vi "产品删除.vi"(8 "error in (no error)":errorcluster caption="错误输入（无错误）") -> (0 "error in (no error) 2":errorcluster caption="错误输入（无错误）")   [LabVIEW 2017]
uses:
  Picture/SaveButtom.ctl
  Global System.vi
panel:
  out "路径输出":path
  out "添加的路径":path
  in  "Vision Paramter Save Buttom":T1
  out "system time":string
  in  "取消按钮":bool
  in  "执行按钮":bool
  in  "原有产品型号":string(combo)
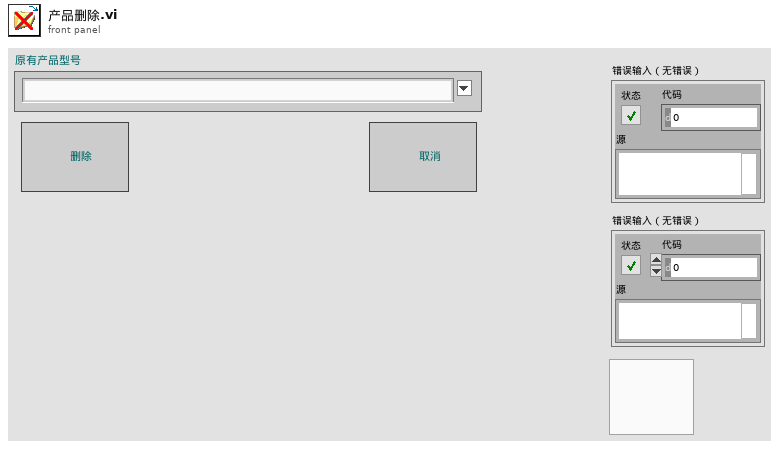
[diagram p1: front panel]
types:
  T1 = typedef "SaveButtom.ctl" = bool
  T2 = cluster{"index":i32, "this vi":refnum<vi>, "error out":errorcluster}
  T3 = cluster{"master data":string, "priority":u16, "secondary data":string[]}
  T4 = cluster{"case name":string[], "queue array":refnum<queue>[]}
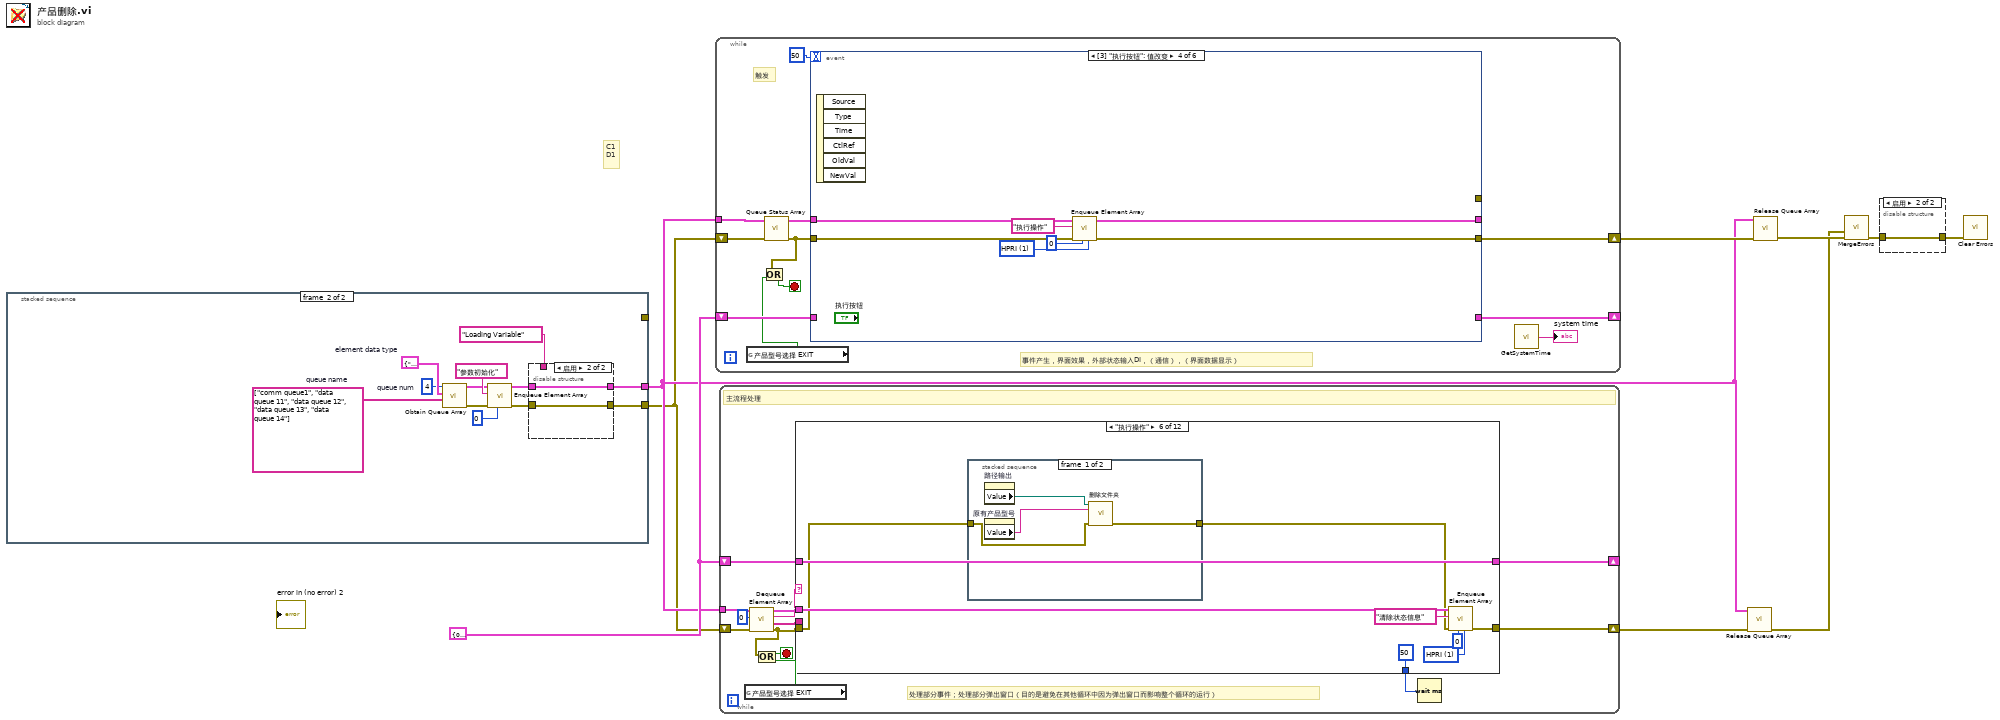
[diagram p0: block diagram]
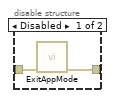
[diagram p2: hidden frame]
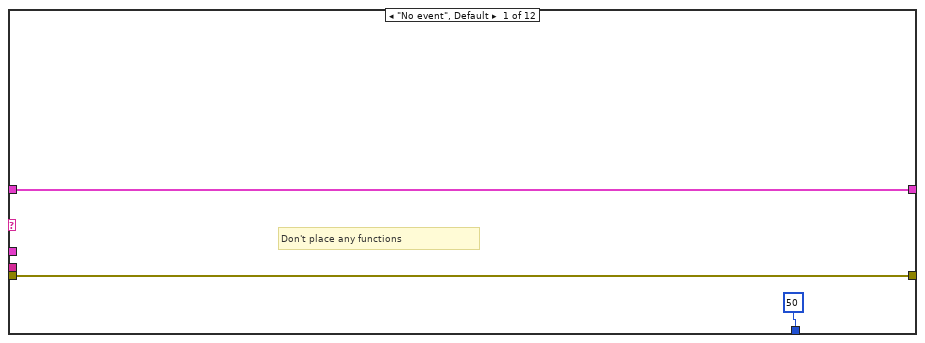
[diagram p3: hidden frame]
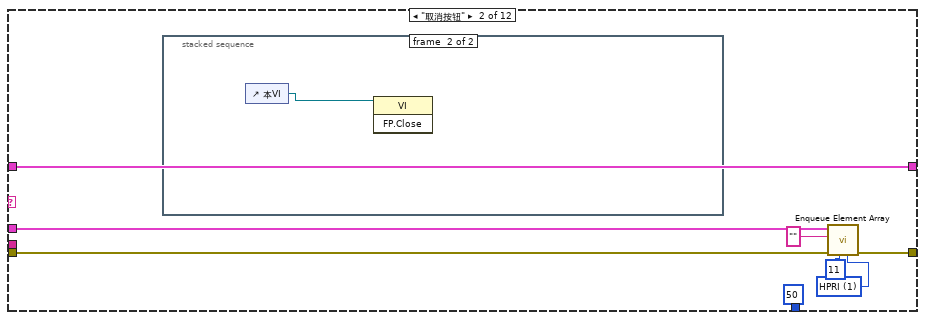
[diagram p4: hidden frame]
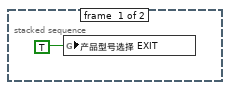
[diagram p5: hidden frame]
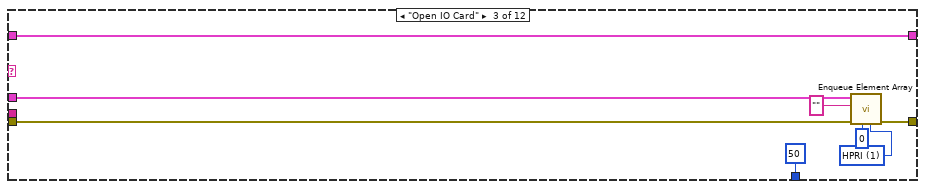
[diagram p6: hidden frame]
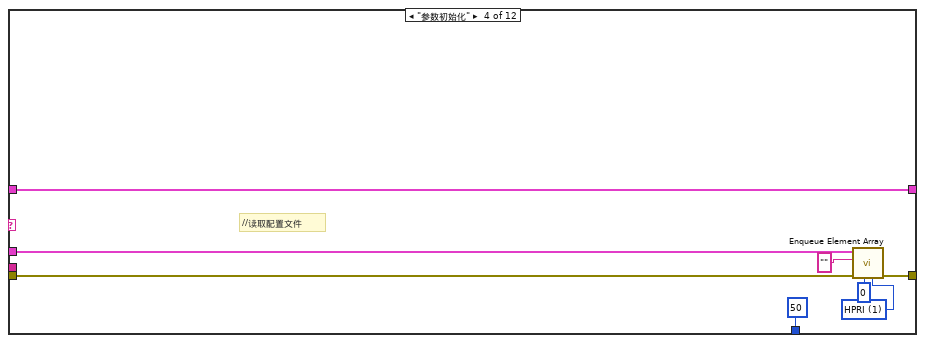
[diagram p7: hidden frame]
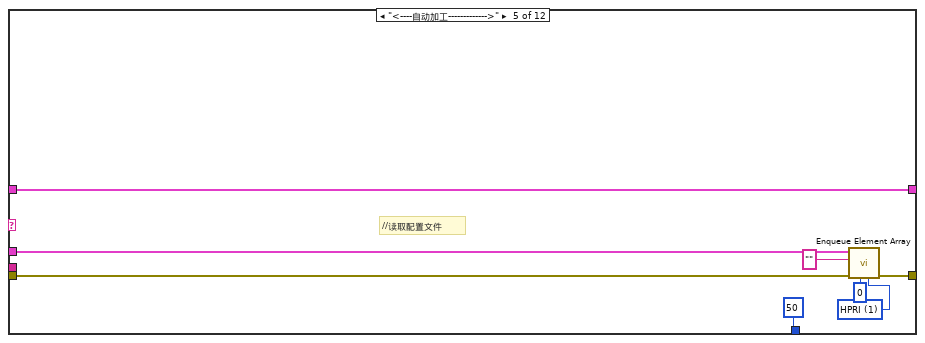
[diagram p8: hidden frame]
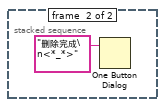
[diagram p9: hidden frame]
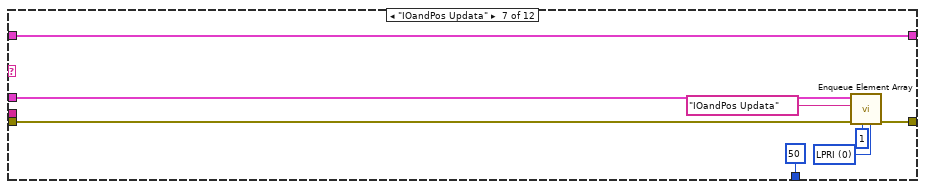
[diagram p10: hidden frame]
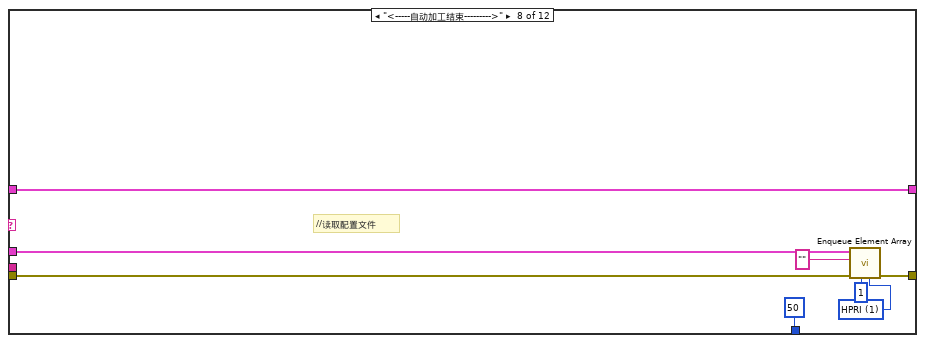
[diagram p11: hidden frame]
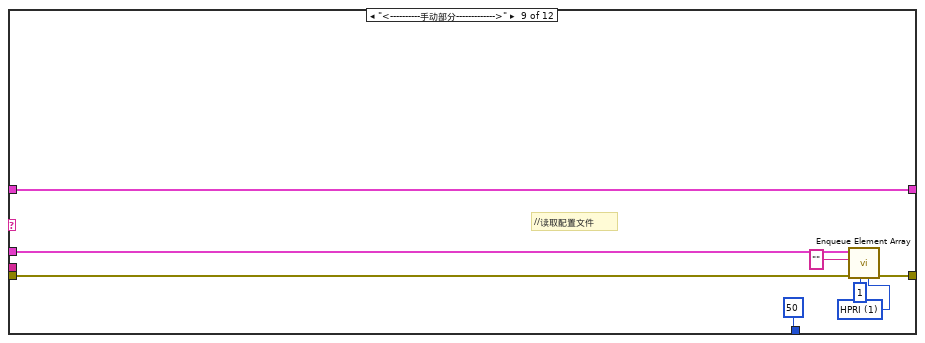
[diagram p12: hidden frame]
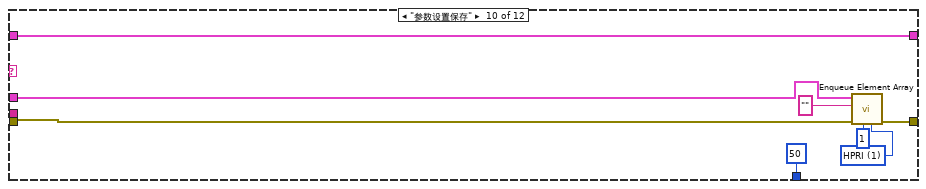
[diagram p13: hidden frame]
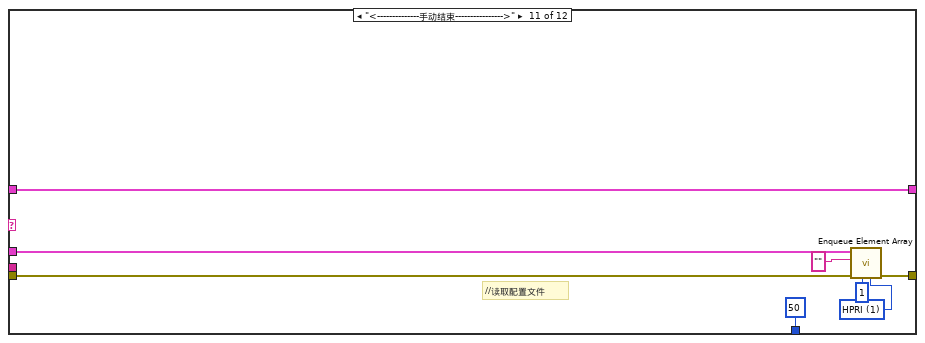
[diagram p14: hidden frame]
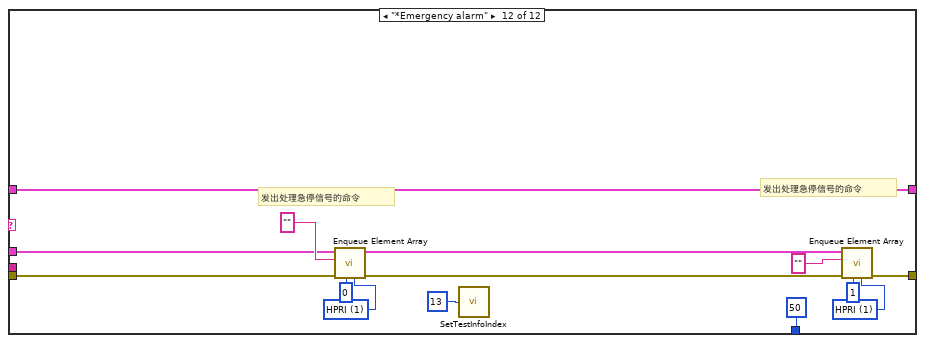
[diagram p15: hidden frame]
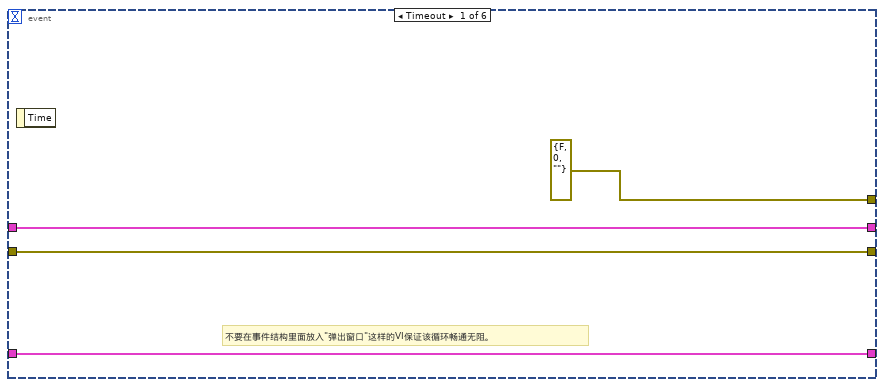
[diagram p16: hidden frame]
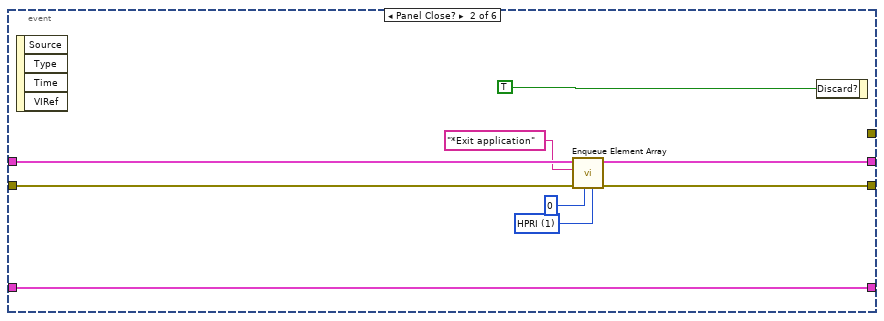
[diagram p17: hidden frame]
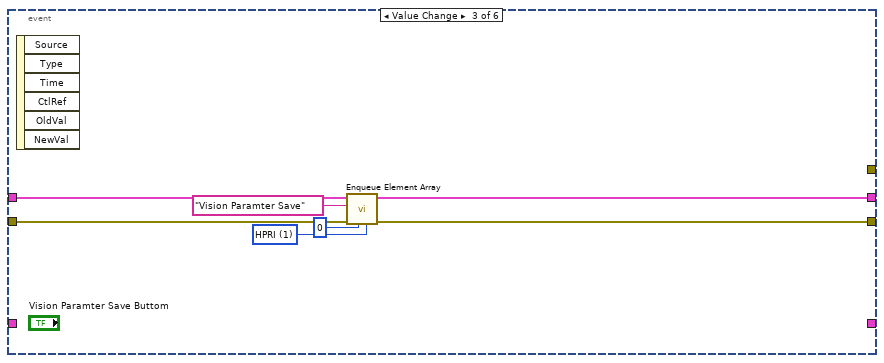
[diagram p18: hidden frame]
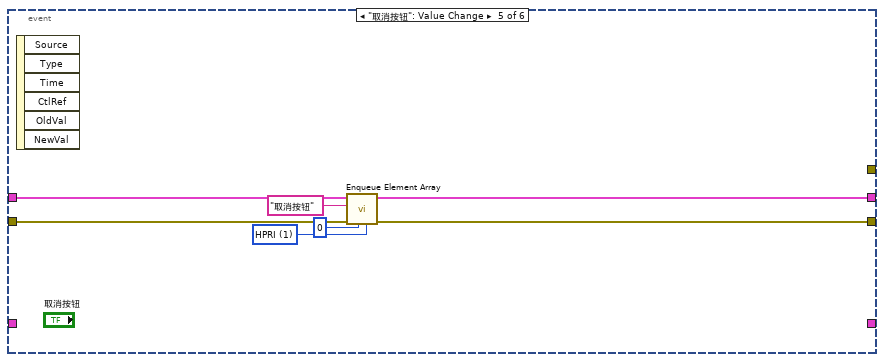
[diagram p19: hidden frame]
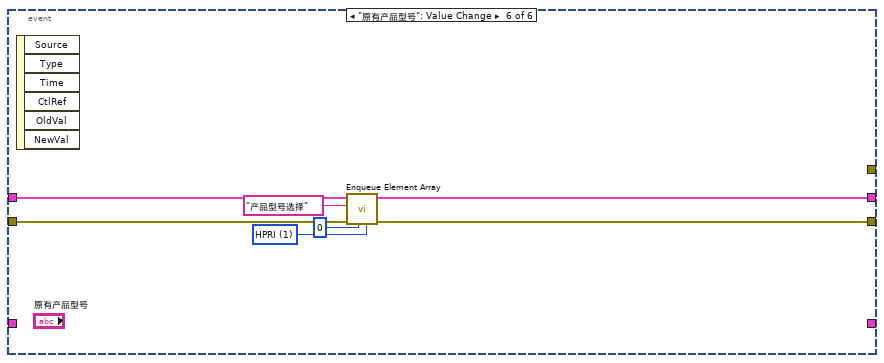
[diagram p20: hidden frame]
diagram:
  w5 = T2 {"index"=0, "this vi"=refnum, "error out"={"status"=FALSE, "code"=0, "source"=""}} ("parameter buffer")
  # "C1\nD1"
  n1 = stacked-sequence {
    tunnel: [w12 _] -> _
    tunnel: [_ w18] -> w1
    tunnel: [_ w17] -> w2
    frame #0 {
      n2 = global write "Global System.vi" "A1 EXIT"(FALSE ("A1 EXIT")) -> ()
      n3 = global read "Global System.vi" "ref path"() -> (w13:path)
      n4 = Build Path(base path=w13, name or relative path="Template Program" ("名称或相对路径")) -> (appended path=w15:path)
      "添加的路径" <- w15
      n5 = List Folder(path=w15) -> (path out=→"路径输出":path, folder names=w16:string[], error out=w12:errorcluster)  [unwired: 3 in, 1 out]
      n6 = property on="原有产品型号" class="CmbBox"("Strings[]"=w16) -> ()  [unwired: 2 in, 2 out]
    }
    frame #1 {
      w26 = string[] ["comm queue1", "data queue 11", "data queue 12", "data queue 13", "data queue 14"]  # queue name
      w27 = 4  # queue num
      w28 = T3 {"master data"="", "priority"=0, "secondary data"=[]}  # element data type
      n7 = call "Obtain Queue Array.vi"("queue name"=w26, "element data type"=w28, "queue num"=w27) -> ("error out"=w22:errorcluster, "queue out"=w23:T4)  [unwired: 2 in, 1 out]
      n8 = call "Enqueue Element Array.vi"("queue index"=0, "error in"=w22, "master data"="参数初始化", "queue in"=w23) -> ("error out"=w21:errorcluster, "queue out"=w20:T4)  [unwired: 6 in]
      n9 = disable-structure shown="启用" {
        disable-tunnel: w21 -> [w34 w35]
        disable-tunnel: w20 -> [w33 w36]
        disable-tunnel: "Loading Variable" ("master data") -> [w32 _]
        disable-tunnel: [w30 w35] -> w18
        disable-tunnel: [w29 w36] -> w17
        frame Disabled {
          n10 = call "Enqueue Element Array.vi"("queue index"=12, "error in"=w34, "master data"=w32, "queue in"=w33) -> ("error out"=w30:errorcluster, "queue out"=w29:T4)  [unwired: 6 in]
        }
        frame Enabled {
        }
      }
    }
  }
  n11 = while {
    shift-right: [w40] -> w6
    shift-left: w1 -> [w44]
    shift-right: [w42] -> _
    shift-left: w5 -> [w43]
    tunnel: w2 -> [w46]
    stop <- w37 stop-if-true
    # "触发"
    # "事件产生，界面效果，外部状态输入DI，（通信），（界面数据显示）"
    n12 = global read "Global System.vi" "产品型号选择 EXIT"() -> (w38:bool)
    n13 = call "Queue Status Array.vi"("error in (no error)"=w44, "queue in"=w46) -> ("error out"=w39:errorcluster, "queue out"=w41:T4)  [unwired: 4 in]
    n14 = Or(x=w39, y=w38) -> (x .or. y?=w37:bool)
    n15 = event shown="[3] \"执行按钮\": 值改变" {
      selector: _ -> [_ _ _ _ _ _]
      dyn-events: _ -> [_ _ _ _ _ _]
      timeout: 50 -> [_ _ _ _ _ _]
      tunnel: w43 -> [w51 w59 _ _ _ _]
      tunnel: [w51 w59 _ _ _ _] -> w42
      tunnel: [errorcluster {"status"=FALSE, "code"=0, "source"=""} ("error out") _ _ _ _ _] -> _
      tunnel: w41 -> [w49 w58 w64 w71 w78 w85]
      tunnel: w39 -> [w48 w57 w63 w70 w77 w84]
      tunnel: [w48 w56 w61 w68 w75 w82] -> w40
      tunnel: [w49 w55 w62 w69 w76 w83] -> _
      event Timeout {
        # "不要在事件结构里面放入\"弹出窗口\"这样的VI保证该循环畅通无阻。"
        n16 = event-data() -> ()  [unwired: 1 in, 1 out]
      }
      event Panel Close? {
        w53 = u16 1 items=["HPRI"=1, "LPRI"=0] ("priority")
        n17 = event-data() -> ()  [unwired: 1 in, 4 out]
        n18 = call "Enqueue Element Array.vi"("priority"=w53, "queue index"=0, "error in"=w57, "master data"="*Exit application", "queue in"=w58) -> ("error out"=w56:errorcluster, "queue out"=w55:T4)  [unwired: 5 in]
        n19 = event-data("Discard?"=TRUE) -> ()  [unwired: 1 in, 1 out]
      }
      event Value Change {
        w66 = u16 1 items=["HPRI"=1, "LPRI"=0] ("priority")
        n20 = event-data() -> ()  [unwired: 1 in, 6 out]
        n21 = call "Enqueue Element Array.vi"("priority"=w66, "queue index"=0, "error in"=w63, "master data"="Vision Paramter Save", "queue in"=w64) -> ("error out"=w61:errorcluster, "queue out"=w62:T4)  [unwired: 5 in]
      }
      event "执行按钮": Value Change {
        w73 = u16 1 items=["HPRI"=1, "LPRI"=0] ("priority")
        n22 = event-data() -> ()  [unwired: 1 in, 6 out]
        n23 = call "Enqueue Element Array.vi"("priority"=w73, "queue index"=0, "error in"=w70, "master data"="执行操作", "queue in"=w71) -> ("error out"=w68:errorcluster, "queue out"=w69:T4)  [unwired: 5 in]
      }
      event "取消按钮": Value Change {
        w80 = u16 1 items=["HPRI"=1, "LPRI"=0] ("priority")
        n24 = event-data() -> ()  [unwired: 1 in, 6 out]
        n25 = call "Enqueue Element Array.vi"("priority"=w80, "queue index"=0, "error in"=w77, "master data"="取消按钮", "queue in"=w78) -> ("error out"=w75:errorcluster, "queue out"=w76:T4)  [unwired: 5 in]
      }
      event "原有产品型号": Value Change {
        w87 = u16 1 items=["HPRI"=1, "LPRI"=0] ("priority")
        n26 = event-data() -> ()  [unwired: 1 in, 6 out]
        n27 = call "Enqueue Element Array.vi"("priority"=w87, "queue index"=0, "error in"=w84, "master data"="产品型号选择", "queue in"=w85) -> ("error out"=w82:errorcluster, "queue out"=w83:T4)  [unwired: 5 in]
      }
    }
    n28 = call "GetSystemTime.vi"() -> ("date/time string"=→"system time":string)  [unwired: 7 in]
  }
  n29 = while {
    shift-right: [w101] -> w4
    shift-left: w1 -> [w92]
    shift-right: [w98] -> _
    shift-left: w5 -> [w99]
    tunnel: w2 -> [w94]
    stop <- w89 stop-if-true
    # "处理部分事件；处理部分弹出窗口（目的是避免在其他循环中因为弹出窗口而影响整个循环的运行）"
    # "主流程处理"
    n30 = global read "Global System.vi" "产品型号选择 EXIT"() -> (w90:bool)
    n31 = call "Dequeue Element Array.vi"("queue in"=w94, "queue index"=0, "error in"=w92) -> ("queue out"=w97:T4, "master data"=w96:string, "secondary data"=w95:string[], "error out"=w91:errorcluster)  [unwired: 2 in, 1 out]
    n32 = Or(x=w91, y=w90) -> (x .or. y?=w89:bool)
    n33 = case shown="\"执行操作\"" w96 {
      tunnel: w97 -> [_ w111 w121 w129 w137 w141 w159 w167 w175 w183 w191 w197]
      tunnel: w91 -> [w103 w107 w117 w126 w133 w140 w154 w163 w171 w179 w187 w194]
      tunnel: [w103 w110 w120 w128 w136 w146 w158 w166 w174 w182 w190 w205] -> w101
      tunnel: [50 50 50 50 50 50 50 50 50 50 50 50] -> w100
      tunnel: w99 -> [w104 w108 w118 w123 w134 w142 w153 w164 w172 w180 w188 w203]
      tunnel: [w104 w108 w118 w123 w134 w142 w153 w164 w172 w180 w188 w203] -> w98
      tunnel: w95 -> [_ _ _ _ _ _ _ _ _ _ _ _]
      frame "No event", Default {
        # "Don't place any functions"
      }
      frame "取消按钮" {
        w105 = u16 1 items=["HPRI"=1, "LPRI"=0] ("priority")
        n34 = stacked-sequence {
          frame #0 {
            n35 = global write "Global System.vi" "产品型号选择 EXIT"(TRUE ("EXIT")) -> ()
          }
          frame #1 {
            n36 = control-ref of="本VI"() -> (w114:refnum<vi>)
            n37 = invoke class="VI" method="FP.Close"(reference=w114) -> ()  [unwired: 2 in, 3 out]
          }
        }
        n38 = call "Enqueue Element Array.vi"("priority"=w105, "queue index"=11, "error in"=w107, "master data"="" ("Element 1"), "queue in"=w111) -> ("error out"=w110:errorcluster)  [unwired: 5 in, 1 out]
      }
      frame "Open IO Card" {
        w115 = u16 1 items=["HPRI"=1, "LPRI"=0] ("priority")
        n39 = call "Enqueue Element Array.vi"("priority"=w115, "queue index"=0, "error in"=w117, "master data"="" ("Element 1"), "queue in"=w121) -> ("error out"=w120:errorcluster)  [unwired: 5 in, 1 out]
      }
      frame "参数初始化" {
        w124 = u16 1 items=["HPRI"=1, "LPRI"=0] ("priority")
        # "//读取配置文件"
        n40 = call "Enqueue Element Array.vi"("priority"=w124, "queue index"=0, "error in"=w126, "master data"="" ("Element 1"), "queue in"=w129) -> ("error out"=w128:errorcluster)  [unwired: 5 in, 1 out]
      }
      frame "<----自动加工------------->" {
        w131 = u16 1 items=["HPRI"=1, "LPRI"=0] ("priority")
        # "//读取配置文件"
        n41 = call "Enqueue Element Array.vi"("priority"=w131, "queue index"=0, "error in"=w133, "master data"="" ("Element 1"), "queue in"=w137) -> ("error out"=w136:errorcluster)  [unwired: 5 in, 1 out]
      }
      frame "执行操作" {
        w143 = u16 1 items=["HPRI"=1, "LPRI"=0] ("priority")
        n42 = stacked-sequence {
          tunnel: w140 -> [w149 _]
          tunnel: [w148 _] -> w139
          frame #0 {
            n43 = property on="路径输出" class="Path"() -> ("Value"=w151:path)  [unwired: 2 in, 2 out]
            n44 = property on="原有产品型号" class="CmbBox"() -> ("Value"=w150:string)  [unwired: 2 in, 2 out]
            n45 = call "删除文件夹.vi"("产品型号路径"=w151, "产品型号"=w150, "error in (no error)"=w149) -> ("error out"=w148:errorcluster)  [unwired: 12 in]
          }
          frame #1 {
            n46 = One Button Dialog(message="删除完成\n<*_*>" ("消息")) -> ()  [unwired: 1 in, 1 out]
          }
        }
        n47 = call "Enqueue Element Array.vi"("priority"=w143, "queue index"=0, "error in"=w139, "master data"="清除状态信息" ("Element 1"), "queue in"=w141) -> ("error out"=w146:errorcluster)  [unwired: 5 in, 1 out]
      }
      frame "IOandPos Updata" {
        w156 = u16 0 items=["HPRI"=1, "LPRI"=0] ("priority")
        n48 = call "Enqueue Element Array.vi"("priority"=w156, "queue index"=1, "error in"=w154, "master data"="IOandPos Updata", "queue in"=w159) -> ("error out"=w158:errorcluster)  [unwired: 5 in, 1 out]
      }
      frame "<-----自动加工结束--------->" {
        w161 = u16 1 items=["HPRI"=1, "LPRI"=0] ("priority")
        # "//读取配置文件"
        n49 = call "Enqueue Element Array.vi"("priority"=w161, "queue index"=1, "error in"=w163, "master data"="" ("Element 1"), "queue in"=w167) -> ("error out"=w166:errorcluster)  [unwired: 5 in, 1 out]
      }
      frame "<----------手动部分------------->" {
        w169 = u16 1 items=["HPRI"=1, "LPRI"=0] ("priority")
        # "//读取配置文件"
        n50 = call "Enqueue Element Array.vi"("priority"=w169, "queue index"=1, "error in"=w171, "master data"="" ("Element 1"), "queue in"=w175) -> ("error out"=w174:errorcluster)  [unwired: 5 in, 1 out]
      }
      frame "参数设置保存" {
        w177 = u16 1 items=["HPRI"=1, "LPRI"=0] ("priority")
        n51 = call "Enqueue Element Array.vi"("priority"=w177, "queue index"=1, "error in"=w179, "master data"="" ("Element 1"), "queue in"=w183) -> ("error out"=w182:errorcluster)  [unwired: 5 in, 1 out]
      }
      frame "<--------------手动结束---------------->" {
        w185 = u16 1 items=["HPRI"=1, "LPRI"=0] ("priority")
        # "//读取配置文件"
        n52 = call "Enqueue Element Array.vi"("priority"=w185, "queue index"=1, "error in"=w187, "master data"="" ("Element 1"), "queue in"=w191) -> ("error out"=w190:errorcluster)  [unwired: 5 in, 1 out]
      }
      frame "*Emergency alarm" {
        w200 = u16 1 items=["HPRI"=1, "LPRI"=0] ("priority")
        w201 = u16 1 items=["HPRI"=1, "LPRI"=0] ("priority")
        # "发出处理急停信号的命令"
        # "发出处理急停信号的命令"
        n53 = call "Enqueue Element Array.vi"("priority"=w200, "queue index"=0, "error in"=w194, "master data"="" ("Element 1"), "queue in"=w197) -> ("error out"=w195:errorcluster, "queue out"=w196:T4)  [unwired: 5 in]
        n54 = call "SetTestInfoIndex.vi"("test info index"=13) -> ()
        n55 = call "Enqueue Element Array.vi"("priority"=w201, "queue index"=1, "error in"=w195, "master data"="" ("Element 1"), "queue in"=w196) -> ("error out"=w205:errorcluster)  [unwired: 5 in, 1 out]
      }
    }
    n56 = Wait (ms)(milliseconds to wait=w100) -> ()  [unwired: 1 out]
  }
  n57 = call "Release Queue Array.vi"("error in"=w4, "queue in"=w2) -> ("error out"=w3:errorcluster)  [unwired: 2 in, 3 out]
  n58 = call "Release Queue Array.vi"("error in"=w6, "queue in"=w2) -> ("error out"=w9:errorcluster)  [unwired: 2 in, 3 out]
  n59 = call "MergeErrors.vi"("error in 3 (no error)"=w3, "error in 4 (no error)"=w9) -> ("error out"=w8:errorcluster)  [unwired: 6 in]
  n60 = disable-structure shown="启用" {
    disable-tunnel: w8 -> [w208 w209]
    disable-tunnel: [w207 w209] -> w7
    frame Disabled {
      n61 = call "ExitAppMode.vi"("error in (no error)"=w208) -> ("error out"=w207:errorcluster)  [unwired: 10 in]
    }
    frame Enabled {
    }
  }
  n62 = call <vilib>:"Clear Errors.vi"("error in (no error)"=w7) -> ()  [unwired: 5 in, 2 out]
